vi "CommonVIs_TimingLogger2.vi"(10 "error in (no error)":errorcluster, 11 "Name":string) -> (2 "error out":errorcluster)   [LabVIEW 2020]
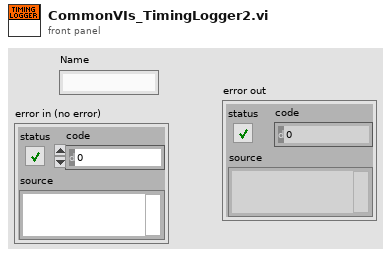
[diagram p1: front panel]
types:
  T1 = enum16{"open", "replace", "create", "open or create", "replace or create", "replace or create with confirmation"}
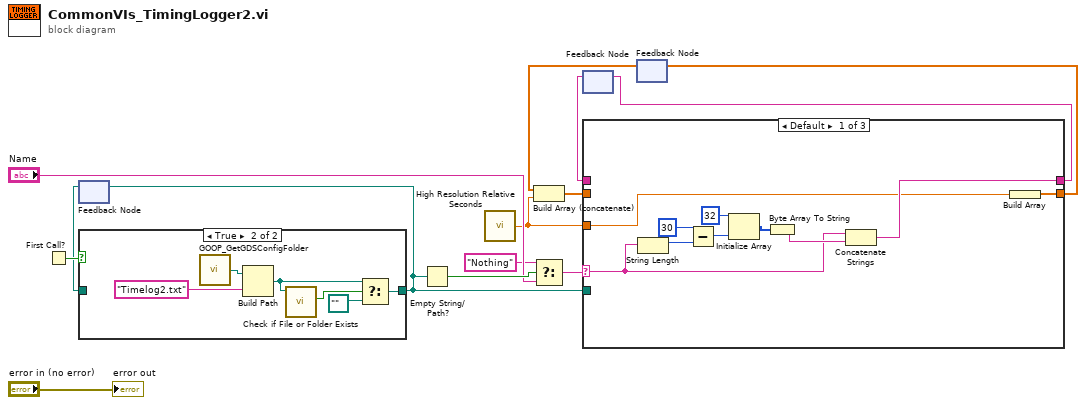
[diagram p0: block diagram]
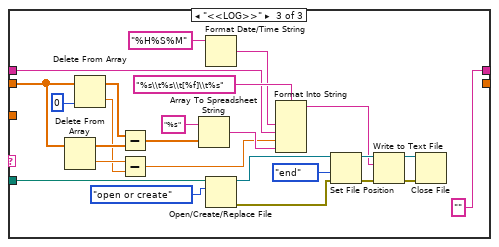
[diagram p4: hidden frame]
diagram:
  n1 = First Call?() -> (First Call?: T/F=w12:bool)
  n2 = feedback #1() -> (w11:path)  [unwired: 1 in]
  n3 = case shown="True" w12 {
    tunnel: [w15 w16] -> w10
    tunnel: w11 -> [w15 _]
    frame False {
    }
    frame True {
      n4 = call <resource>:"GOOP_GetGDSConfigFolder.vi"() -> ("GDSFolderPath"=w21:path)
      n5 = Build Path(base path=w21, name or relative path="Timelog2.txt") -> (appended path=w17:path)
      n6 = call <vilib>:"Check if File or Folder Exists.vi"("path"=w17) -> ("file or folder exists?"=w19:bool)  [unwired: 8 in, 2 out]
      n7 = Select(t=w17, s=w19, f=path "") -> (s? t:f=w16:path)
    }
  }
  n8 = feedback-in #1(w10) -> ()
  n9 = Empty String/Path?(string/path=w10) -> (empty?=w9:bool)
  n10 = call <vilib>:"High Resolution Relative Seconds.vi"() -> ("relative seconds"=w1:dbl)
  n11 = Select(t="Nothing", s=w9, f="Name") -> (s? t:f=w7:string)
  n12 = feedback #2() -> (w13:string)  [unwired: 1 in]
  n13 = feedback #3() -> (w5:dbl[])  [unwired: 1 in]
  n14 = Build Array (concatenate)(w5, w1) -> (w4:dbl[])
  n15 = case shown="Default" w7 {
    selector: w7 -> [w25 _ _]
    tunnel: [w24 w33 ""] -> w14
    tunnel: w13 -> [_ w33 w36]
    tunnel: w4 -> [_ w32 w41]
    tunnel: [w23 w32 _] -> w3
    tunnel: w10 -> [_ _ w34]
    tunnel: w1 -> [w22 _ _]
    frame Default {
      n16 = String Length(string=w25) -> (length=w31:i32)
      n17 = Subtract(x=30, y=w31) -> (x-y=w29:i32)
      n18 = Initialize Array(u8 32 ("element"), w29) -> (w27:u8[])
      n19 = Byte Array To String(unsigned byte array=w27) -> (string=w26:string)
      n20 = Concatenate Strings(w25, w26) -> (w24:string)
      n21 = Build Array(w22) -> (w23:dbl[])
    }
    frame "" {
    }
    frame "<<LOG>>" {
      n22 = Delete From Array(array=w41) -> (deleted portion=w38:dbl, array with subset deleted=w40:dbl[])  [unwired: 2 in]
      n23 = Delete From Array(array=w41, index=0) -> (deleted portion=w37:dbl, array with subset deleted=w39:dbl[])  [unwired: 1 in]
      n24 = Subtract(x=w39, y=w40) -> (x-y=w55:dbl[])
      n25 = Subtract(x=w38, y=w37) -> (x-y=w35:dbl)
      n26 = Array To Spreadsheet String(array=w55, 3:"%s" ("format string")) -> (spreadsheet string=w52:string)  [unwired: 1 in]
      n27 = Format Date/Time String(time format string (%c)="%H%S%M") -> (date/time string=w53:string)  [unwired: 2 in]
      n28 = Open/Create/Replace File(file path (use dialog)=w34, operation (0:open)=T1."open or create") -> (refnum out=w50:refnum<file>, error out=w49:errorcluster)  [unwired: 4 in, 1 out]
      n29 = Format Into String(format string="%s\\t%s\\t[%f]\\t%s", w53, w36, w35, w52) -> (resulting string=w45:string)  [unwired: 2 in, 1 out]
      n30 = Set File Position(refnum=w50, from (0:start)=enum16{"start", "end", "current"}."end", error in=w49) -> (refnum out=w47:refnum<file>, error out=w46:errorcluster)  [unwired: 1 in]
      n31 = Write to Text File(file (use dialog)=w47, text=w45, error in=w46) -> (refnum out=w43:refnum<file>, error out=w44:errorcluster)  [unwired: 1 in, 1 out]
      n32 = Close File(refnum=w43, error in=w44) -> ()  [unwired: 2 out]
    }
  }
  n33 = feedback-in #2(w14) -> ()
  n34 = feedback-in #3(w3) -> ()
  "error out" <- "error in (no error)"
